vi "Proyecto llenado y vaciado de un tanque.vi"() -> ()   [LabVIEW 2020]
panel:
  in  "stop 2":bool
  in  "stop":bool
  out "TANQUE VACIO":bool
  out "TANQUE MEDIO":bool
  out "Tank":dbl(slide) scale=0.0..100.0
  out "TANQUE LLENO":bool
  out "Boolean 4":bool
  out "Boolean 3":bool
  in  "VACIADO DEL TANQUE":bool
  in  "LLENADO DEL TANQUE":bool
  out "MEDIDOR":dbl(knob) scale=0.0..100.0
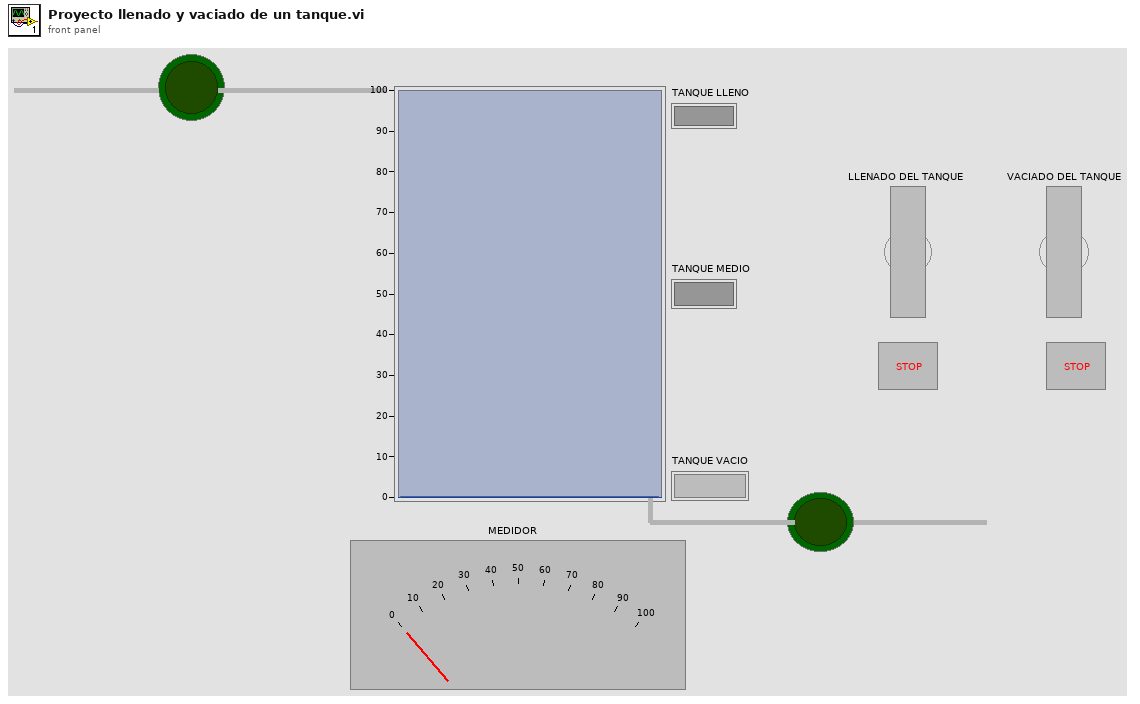
[diagram p1: front panel]
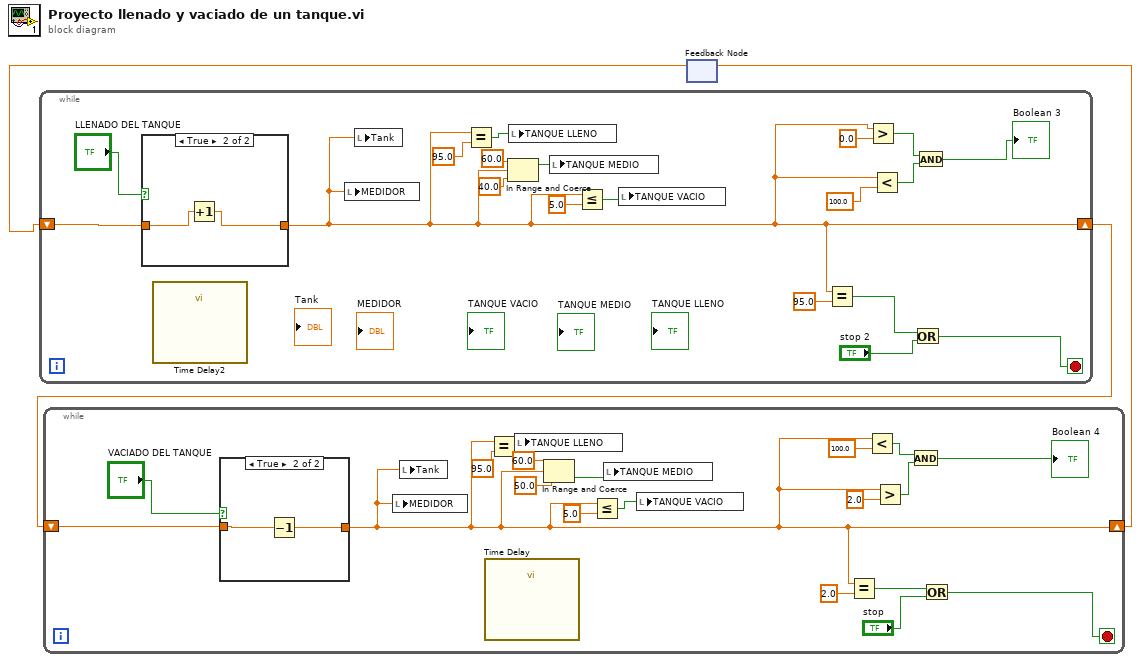
[diagram p0: block diagram]
diagram:
  n1 = feedback #1() -> (w1:dbl)  [unwired: 1 in]
  n2 = while {
    shift-right: [w7] -> w3
    shift-left: w1 -> [w21]
    stop <- w4 stop-if-true
    n3 = case shown="True" "LLENADO DEL TANQUE" {
      tunnel: w21 -> [w23 w25]
      tunnel: [w23 w24] -> w7
      frame False {
      }
      frame True {
        n4 = Increment(x=w25) -> (x+1=w24:dbl)
      }
    }
    n5 = call "Time Delay2"() -> ()  [unwired: 11 in, 1 out]
    n6 = local write "MEDIDOR"(w7) -> ()
    n7 = local write "Tank"(w7) -> ()
    n8 = Equal?(x=w7, y=95.0) -> (x = y?=w19:bool)
    n9 = In Range and Coerce(upper limit=60.0 ("x"), x=w7, lower limit=40.0 ("y")) -> (In Range?=w10:bool)  [unwired: 1 out]
    n10 = local write "TANQUE LLENO"(w19) -> ()
    n11 = local write "TANQUE MEDIO"(w10) -> ()
    n12 = Less Or Equal?(x=w7, y=5.0) -> (x <= y?=w18:bool)
    n13 = local write "TANQUE VACIO"(w18) -> ()
    n14 = Equal?(x=w7, y=95.0) -> (x = y?=w6:bool)
    n15 = Greater?(x=w7, y=0.0) -> (0:w14:bool)
    n16 = Less?(x=w7, y=100.0 ("x")) -> (x < y?=w13:bool)
    n17 = Or(x=w6, y="stop 2") -> (x .or. y?=w4:bool)
    n18 = And(x=w14, y=w13) -> (x .and. y?=→"Boolean 3":bool)
  }
  n19 = while {
    shift-right: [w29] -> w2
    shift-left: w3 -> [w43]
    stop <- w27 stop-if-true
    n20 = case shown="True" "VACIADO DEL TANQUE" {
      tunnel: w43 -> [w45 w47]
      tunnel: [w45 w46] -> w29
      frame False {
      }
      frame True {
        n21 = Decrement(x=w47) -> (x-1=w46:dbl)
      }
    }
    n22 = local write "MEDIDOR"(w29) -> ()
    n23 = local write "Tank"(w29) -> ()
    n24 = call "Time Delay"() -> ()  [unwired: 11 in, 1 out]
    n25 = Equal?(x=w29, y=95.0) -> (x = y?=w41:bool)
    n26 = local write "TANQUE LLENO"(w41) -> ()
    n27 = In Range and Coerce(upper limit=60.0 ("coerced(x)"), x=w29, lower limit=50.0 ("y")) -> (In Range?=w38:bool)  [unwired: 1 out]
    n28 = Less Or Equal?(x=w29, y=5.0) -> (x <= y?=w39:bool)
    n29 = local write "TANQUE MEDIO"(w38) -> ()
    n30 = local write "TANQUE VACIO"(w39) -> ()
    n31 = Equal?(x=w29, y=2.0) -> (x = y?=w28:bool)
    n32 = Less?(x=w29, y=100.0) -> (x < y?=w33:bool)
    n33 = Greater?(x=w29, y=2.0) -> (0:w32:bool)
    n34 = And(x=w33, y=w32) -> (x .and. y?=→"Boolean 4":bool)
    n35 = Or(x=w28, y="stop") -> (x .or. y?=w27:bool)
  }
  n36 = feedback-in #1(w2) -> ()
